vi "09_2.vi"() -> ()   [LabVIEW 2018]
panel:
  out "Part 2":dbl
  in  "length":i32=25
  out "Part 1":dbl=25918798.0
  in  "#Elements":i32=2
  in  "Input":string="14\n9\n43\n18\n13\n24\n3\n38\n33\n8\n41\n4\n32\n15\n31\n44\n17\n34\n21\n10\n50\n37\n2\n23\n6\n47\n5\n9\n11\n16\n12\n18\n7\n13\n26\n14\n19\n8\n20\n15\n29\n58\n17\n22\n21\n24\n25\n10\n27\n31\n33\n23\n28\n30\n34\n32\n35\n38\n49\n18\n26\n36\n37\n47\n39\n56\n40\n42\n43\n41\n44\n45\n46\n48\n50\n51\n53\n79\n73\n69\n117\n54\n55\n90\n57\n62\n75\n114\n85\n94\n110\n81\n98\n153\n86\n89\n204\n96\n101\n103\n104\n152\n169\n124\n135\n109\n143\n171\n119\n132\n137\n207\n166\n167\n184\n185\n170\n175\n182\n187\n190\n197\n233\n204\n212\n244\n299\n228\n339\n241\n246\n269\n415\n319\n298\n349\n337\n333\n444\n357\n345\n362\n365\n562\n377\n387\n401\n416\n541\n469\n472\n474\n647\n591\n487\n515\n567\n617\n686\n1158\n793\n670\n678\n702\n864\n710\n856\n781\n817\n764\n1251\n1214\n885\n941\n943\n..."
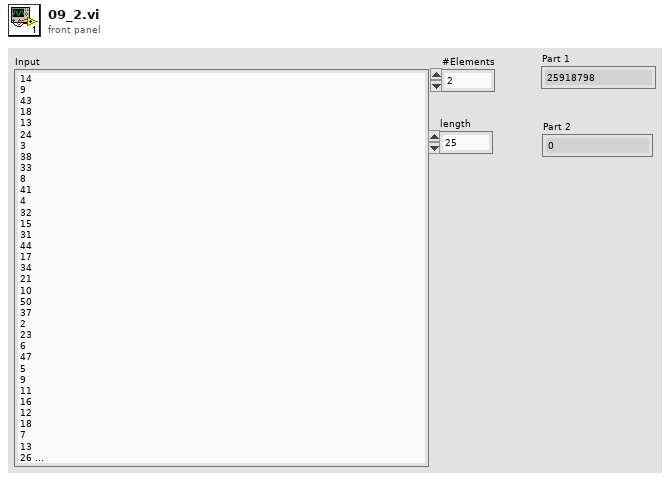
[diagram p1: front panel]
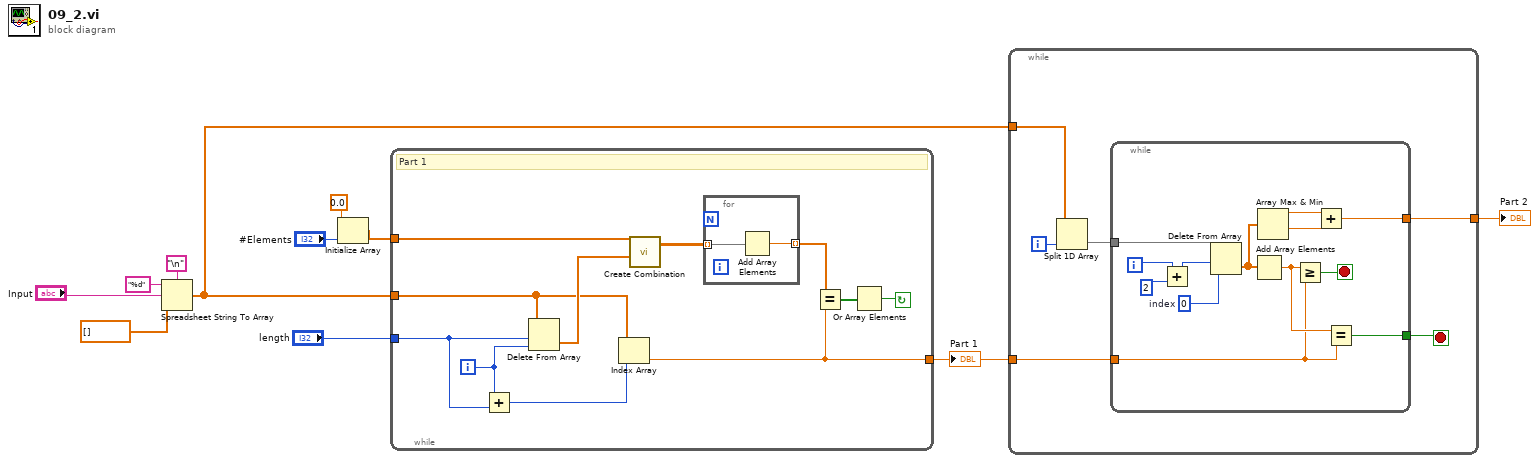
[diagram p0: block diagram]
diagram:
  n1 = Spreadsheet String To Array(delimiter (Tab)="\n", format string="%d", spreadsheet string="Input", array type (2D Dbl)=dbl[] []) -> (array=w1:dbl[])
  n2 = Initialize Array(0.0, "#Elements") -> (w5:dbl[])
  n3 = while {
    tunnel: w5 -> [w22]
    tunnel: w1 -> [w17]
    tunnel: "length" -> [w13]
    tunnel: [w15] -> w3
    i -> [w12]
    stop <- w20 continue-if-true
    # "Part 1"
    n4 = Add(x=w12, y=w13) -> (x+y=w18:i32)
    n5 = Delete From Array(array=w17, length=w13, index=w12) -> (deleted portion=w19:dbl[])  [unwired: 1 out]
    n6 = Index Array(array=w17, index=w18) -> (element=w15:dbl)
    n7 = call "Create Combination.vi"("Array"=w19, "Temp Combination"=w22) -> ("Combinations Out"=w21:dbl[][])  [unwired: 9 in]
    n8 = for {
      tunnel: w21 -> [w24] mode=indexing
      tunnel: [w23] -> w16 mode=indexing
      n9 = Add Array Elements(numeric array=w24) -> (sum=w23:dbl)
    }
    n10 = Equal?(x=w16, y=w15) -> (x = y?=w14:bool[])
    n11 = Or Array Elements(Boolean array=w14) -> (logical OR=w20:bool)
  }
  "Part 1" <- w3
  n12 = while {
    tunnel: w1 -> [w30]
    tunnel: w3 -> [w27]
    tunnel: [w25] -> w2
    i -> [w29]
    stop <- w26 stop-if-true
    n13 = Split 1D Array(array=w30, index=w29) -> (second subarray=w28:dbl[])  [unwired: 1 out]
    n14 = while {
      tunnel: w28 -> [w43]
      tunnel: w27 -> [w37]
      tunnel: [w36] -> w26
      tunnel: [w32] -> w25
      i -> [w41]
      stop <- w39 stop-if-true
      w31 = 0  # index
      n15 = Add(x=w41, y=2) -> (x+y=w40:i32)
      n16 = Delete From Array(array=w43, length=w40, index=w31) -> (deleted portion=w35:dbl[])  [unwired: 1 out]
      n17 = Add Array Elements(numeric array=w35) -> (sum=w38:dbl)
      n18 = Array Max & Min(array=w35) -> (max value=w34:dbl, min value=w33:dbl)  [unwired: 2 out]
      n19 = Greater Or Equal?(x=w38, y=w37) -> (x >= y?=w39:bool)
      n20 = Add(x=w34, y=w33) -> (x+y=w32:dbl)
      n21 = Equal?(x=w38, y=w37) -> (x = y?=w36:bool)
    }
  }
  "Part 2" <- w2
